vi "add_child_queue.vi"(7 "waitgroup":T1, 8 "error in (no error)":errorcluster, 11 "queue":refnum<queue>) -> (0 "error out":errorcluster, 3 "child_id":T2)   [LabVIEW 2015, in "lv-waitgroup.lvlib"]
uses:
  lv-waitgroup.lvlib
  _controls/api_child_queue.ctl
  _controls/api_waitgroup.ctl
  private/_controls/waitgroup.ctl
  _controls/data_error.ctl
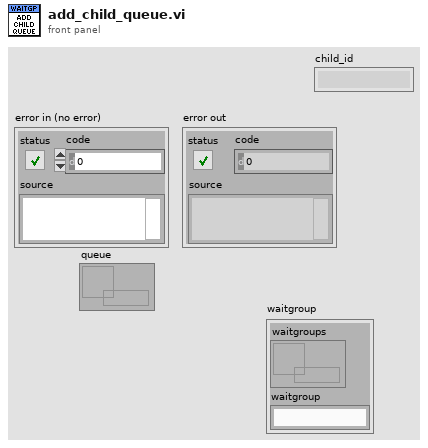
[diagram p1: front panel]
types:
  T1 = typedef "lv-waitgroup.lvlib/api_waitgroup.ctl" = cluster{"waitgroups":refnum<data-value>, "waitgroup":string}
  T2 = typedef "lv-waitgroup.lvlib/api_child_queue.ctl" = string
  T3 = typedef "lv-waitgroup.lvlib/waitgroup.ctl" = cluster{"waitgroup":refnum<queue>, "queues":variant}
  T4 = typedef "lv-waitgroup.lvlib/data_error.ctl" = enum16{"<data_error>", "unable_to_generate_id", "waitgroup_not_found", "unable_to_add_to_waitgroup", "<null>"}
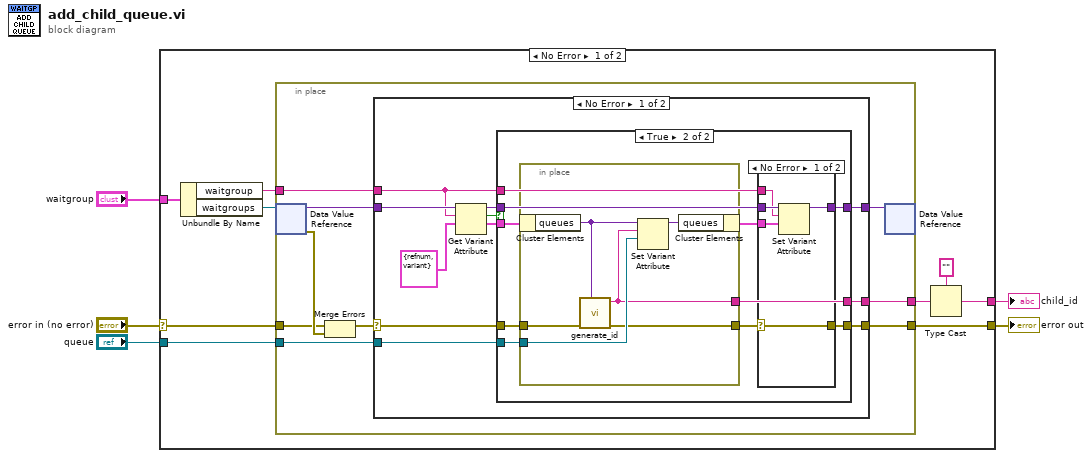
[diagram p0: block diagram]
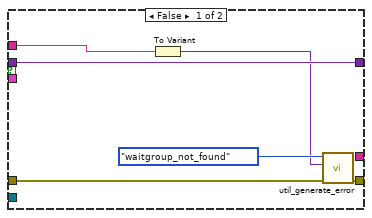
[diagram p2: hidden frame]
diagram:
  n1 = case shown="No Error" "error in (no error)" {
    selector: "error in (no error)" -> [w6 w66]
    tunnel: [w13 w66] -> w5
    tunnel: "waitgroup" -> [w9 _]
    tunnel: "queue" -> [w14 _]
    tunnel: [w12 _] -> w2
    frame No Error {
      n2 = Unbundle By Name(w9) -> ("waitgroup"=w8:string, "waitgroups"=w7:refnum<data-value>)
      n3 = in-place {
        in-place-border: w6 -> [w22]
        in-place-border: w14 -> [w21]
        in-place-border: [w16] -> w13
        in-place-border: w8 -> [w18]
        in-place-border: [w15] -> w10
        n4 = in-place-dvr #1(w7) -> (w20:variant, w23:errorcluster)
        n5 = Merge Errors(w22, w23) -> (w17:errorcluster)
        n6 = case shown="No Error" w17 {
          selector: w17 -> [w27 w65]
          tunnel: w21 -> [w32 _]
          tunnel: w20 -> [w31 w64]
          tunnel: [w30 w64] -> w19
          tunnel: w18 -> [w29 _]
          tunnel: [w26 w65] -> w16
          tunnel: [w25 _] -> w15
          frame No Error {
            n7 = Get Variant Attribute(Variant=w31, name=w29, default value (empty Variant)=T3 {"waitgroup"=refnum, "queues"=variant(refnum<queue>[] [])} ("shared_data")) -> (duplicate Variant=w33:variant, found=w24:bool, value=w28:T3)  [unwired: 1 in, 1 out]
            n8 = case shown="True" w24 {
              tunnel: w33 -> [w40 w50]
              tunnel: w32 -> [_ w49]
              tunnel: [w40 w48] -> w30
              tunnel: w29 -> [w36 w47]
              tunnel: w28 -> [_ w46]
              tunnel: w27 -> [w38 w44]
              tunnel: [w37 w41] -> w26
              tunnel: [_ w43] -> w25
              frame False {
                n9 = To Variant(anything=w36) -> (Variant=w35:variant)
                n10 = call "util_generate_error.vi"("error in (no error)"=w38, "data"=w35, "data_error"=data_error."waitgroup_not_found") -> ("error out"=w37:errorcluster)  [unwired: 8 in]
              }
              frame True {
                n11 = in-place {
                  in-place-border: w44 -> [w63]
                  in-place-border: w49 -> [w62]
                  in-place-border: [w59] -> w42
                  in-place-border: [w58] -> w43
                  n12 = in-place-cluster #2(w46) -> ("queues"=w60:variant)
                  n13 = call "generate_id.vi"("queues"=w60, "error in (no error)"=w63) -> ("error out"=w59:errorcluster, "id"=w58:string)  [unwired: 8 in]
                  n14 = Set Variant Attribute(Variant=w60, name=w58, value=w62) -> (Variant out=w61:variant)  [unwired: 1 in, 2 out]
                  n15 = in-place-cluster #2("queues"=w61) -> (w45:T3)
                }
                n16 = case shown="No Error" w42 {
                  selector: w42 -> [w51 w56]
                  tunnel: w50 -> [w55 w57]
                  tunnel: [w54 w57] -> w48
                  tunnel: w47 -> [w53 _]
                  tunnel: w45 -> [w52 _]
                  tunnel: [w51 w56] -> w41
                  frame No Error {
                    n17 = Set Variant Attribute(Variant=w55, name=w53, value=w52) -> (Variant out=w54:variant)  [unwired: 1 in, 2 out]
                  }
                  frame Error {
                  }
                }
              }
            }
          }
          frame Error {
          }
        }
        n18 = in-place-dvr #1(w19) -> ()  [unwired: 2 out]
      }
      n19 = Type Cast(type=T2 "" ("shared_data"), x=w10) -> (*(type *) &x=w12:T2)
    }
    frame Error {
    }
  }
  "error out" <- w5
  "child_id" <- w2
